vi "Fade For Loop.vi"(8 "error in (no error)":errorcluster, 11 "Array in":refnum<class "Button.lvclass">[](array[class])) -> (0 "error out":errorcluster, 3 "Array out":refnum<class "Button.lvclass">[](array[class]))   [LabVIEW 2019]
uses:
  Button Class/Button.lvclass
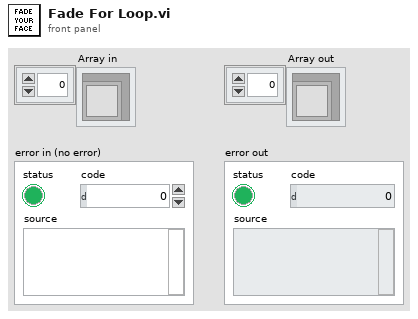
[diagram p1: front panel]
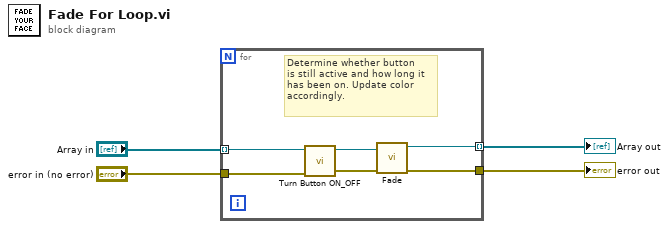
[diagram p0: block diagram]
diagram:
  n1 = for {
    tunnel: "Array in" -> [w8] mode=indexing
    tunnel: [w10] -> w2
    tunnel: [w9] -> w3 mode=indexing
    tunnel: "error in (no error)" -> [w7]
    # "Determine whether button\nis still active and how long it\nhas been on. Update color \naccordingly."
    n2 = call "Turn Button ON_OFF.vi"("error in (no error)"=w7, "Button in"=w8) -> ("error out"=w5:errorcluster, "Button out"=w6:refnum<class "Button.lvclass">)  [unwired: 8 in]
    n3 = call "Fade.vi"("error in (no error)"=w5, "Button in"=w6) -> ("error out"=w10:errorcluster, "Button out"=w9:refnum<class "Button.lvclass">)  [unwired: 8 in]
  }
  "Array out" <- w3
  "error out" <- w2
